vi "p4.2.vi"() -> ()   [LabVIEW 2020]
uses:
  <vilib>/Analysis/2dsp.llb/Upsample (DBL).vi
  <vilib>/Analysis/NI_AALBase.lvlib
  <vilib>/Analysis/NI_AALPro.lvlib
panel:
  out "FFT(Expansor L=3)":dbl[](graph)
  out "FFT(Expansor L=2)":dbl[](graph)
  out "FFT(original)":dbl[](graph)
  in  "L =3":i32=1
  out "Expansor L=3":dbl[](graph)
  out "Expansor L=2":dbl[](graph)
  in  "L=2":i32=1
  out "cos(0,0.3pi) + cos(0,0.4pi) - Original":dbl[](graph)
  in  "Frecuencia cos(0,4pi)":dbl=0.0078125 format="%0.4e"
  out "cos(0,0.4pi)":dbl[](graph)
  out "cos(0,0.3pi)":dbl[](graph)
  in  "Frecuencia cos(0,3pi)":dbl=0.0078125 format="%0.4e"
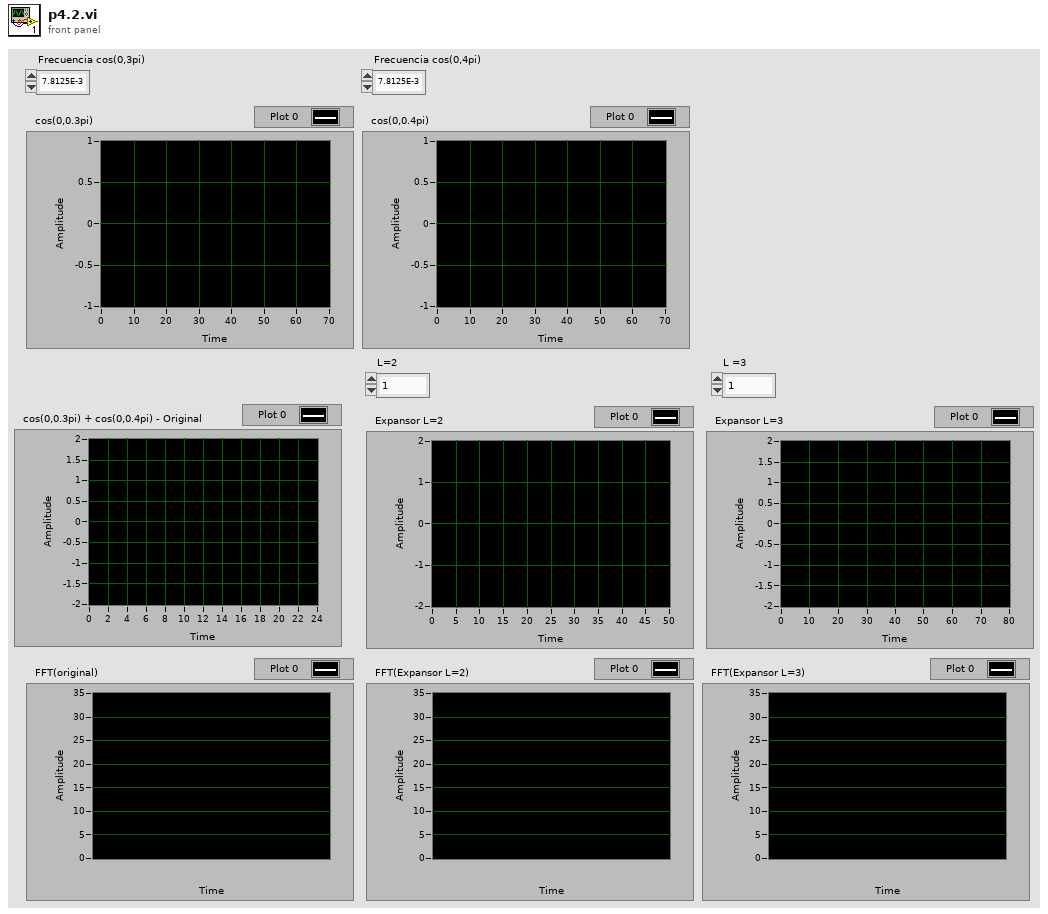
[diagram p1: front panel]
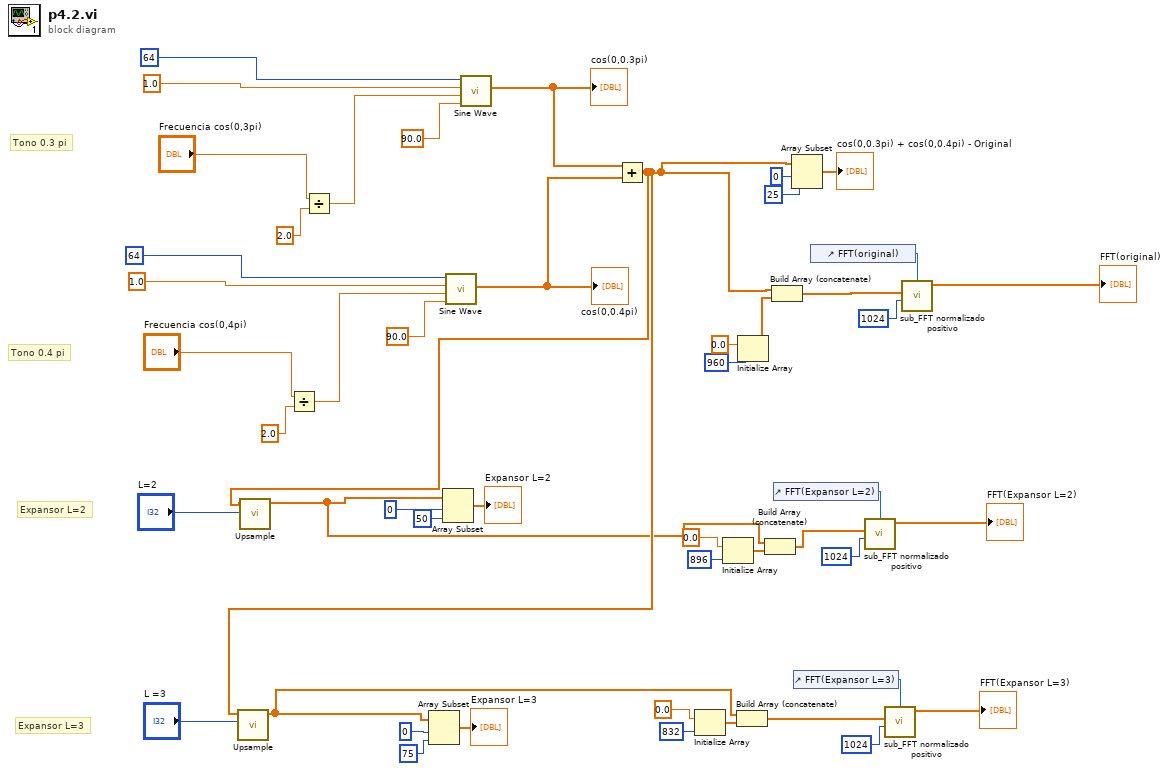
[diagram p0: block diagram]
diagram:
  # "Expansor L=3"
  # "Expansor L=2"
  # "Tono 0.4 pi"
  # "Tono 0.3 pi"
  n1 = Divide(x="Frecuencia cos(0,4pi)", y=2.0) -> (x/y=w42:dbl)
  n2 = Divide(x="Frecuencia cos(0,3pi)", y=2.0) -> (x/y=w45:dbl)
  n3 = call <vilib>:"Sine Wave.vi"("samples"=64, "amplitude"=1.0, "frequency"=w42, "phase in"=90.0) -> ("sine wave"=w36:dbl[])  [unwired: 1 in, 2 out]
  "cos(0,0.4pi)" <- w36
  n4 = call <vilib>:"Sine Wave.vi"("samples"=64, "amplitude"=1.0, "frequency"=w45, "phase in"=90.0) -> ("sine wave"=w37:dbl[])  [unwired: 1 in, 2 out]
  "cos(0,0.3pi)" <- w37
  n5 = Add(x=w37, y=w36) -> (x+y=w12:dbl[])
  n6 = call-poly <vilib>:"Upsample.vi"("upsampling factor"="L =3", "X"=w12) -> ("Upsampled Array"=w2:dbl[])  [unwired: 8 in, 1 out]
  n7 = call-poly <vilib>:"Upsample.vi"("upsampling factor"="L=2", "X"=w12) -> ("Upsampled Array"=w7:dbl[])  [unwired: 8 in, 1 out]
  n8 = Array Subset(array=w2, index=0, length=75) -> (→"Expansor L=3":dbl[])
  n9 = Array Subset(array=w7, index=0, length=50) -> (→"Expansor L=2":dbl[])
  n10 = Initialize Array(0.0 ("element"), 832 ("dimension size")) -> (w3:dbl[])
  n11 = Initialize Array(0.0 ("element"), 896 ("dimension size")) -> (w10:dbl[])
  n12 = Build Array (concatenate)(w2, w3) -> (w1:dbl[])
  n13 = Initialize Array(0.0 ("element"), 960 ("dimension size")) -> (w22:dbl[])
  n14 = Build Array (concatenate)(w7, w10) -> (w6:dbl[])
  n15 = Build Array (concatenate)(w12, w22) -> (w21:dbl[])
  n16 = control-ref of="FFT(Expansor L=2)"() -> (w19:refnum<vi>)
  n17 = Array Subset(array=w12, index=0, length=25) -> (→"cos(0,0.3pi) + cos(0,0.4pi) - Original":dbl[])
  n18 = control-ref of="FFT(Expansor L=3)"() -> (w14:refnum<vi>)
  n19 = control-ref of="FFT(original)"() -> (w20:refnum<vi>)
  n20 = call "sub_FFT normalizado positivo.vi"("FFT size"=1024, "Array in"=w6, "WaveformGraph in"=w19) -> ("Array out"=→"FFT(Expansor L=2)":dbl[])  [unwired: 8 in]
  n21 = call "sub_FFT normalizado positivo.vi"("FFT size"=1024, "Array in"=w1, "WaveformGraph in"=w14) -> ("Array out"=→"FFT(Expansor L=3)":dbl[])  [unwired: 8 in]
  n22 = call "sub_FFT normalizado positivo.vi"("FFT size"=1024, "Array in"=w21, "WaveformGraph in"=w20) -> ("Array out"=→"FFT(original)":dbl[])  [unwired: 8 in]
